vi "Add Headers.vi"(8 "error in (no error)":errorcluster, 10 "headers":cluster{"header":string, "value":string}[](array[cluster]), 11 "HttpHeaders_NET in":refnum<class "HttpHeaders_NET.lvclass">) -> (0 "error out":errorcluster, 3 "HttpHeaders_NET out":refnum<class "HttpHeaders_NET.lvclass">)   [LabVIEW 2018, in "HttpClient_NET.lvlib" / "HttpHeaders_NET.lvclass"]
doc: "<b> </b> <b> </b>\nHttpClient_NET\nJustin Young - Viviota\nCopyright (c) 2021\nLicense: BSD"
uses:
  HttpHeaders_NET.lvclass
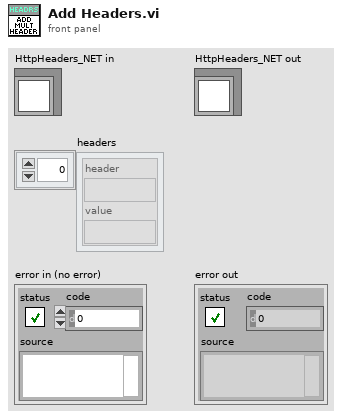
[diagram p1: front panel]
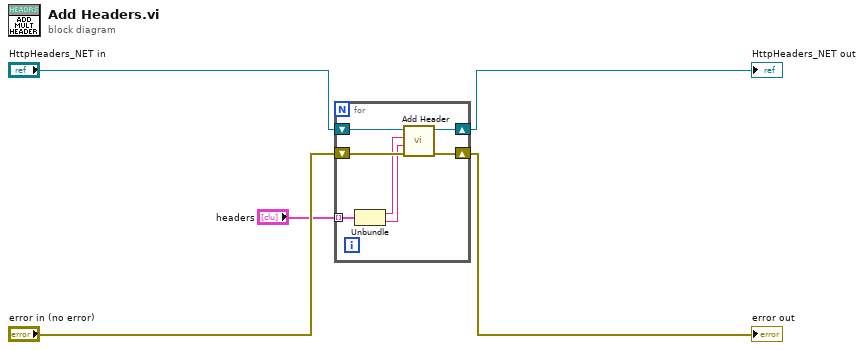
[diagram p0: block diagram]
diagram:
  n1 = for {
    tunnel: "headers" -> [w11] mode=indexing
    shift-right: [w8] -> w4
    shift-left: "HttpHeaders_NET in" -> [w6]
    shift-right: [w7] -> w2
    shift-left: "error in (no error)" -> [w12]
    n2 = Unbundle(w11) -> ("header"=w10:string, "value"=w9:string)
    n3 = call-dynamic "Add Header.vi"("error in (no error)"=w12, "Value"=w9, "Name"=w10, "HTTPHeaders_NET in"=w6) -> ("error out"=w7:errorcluster, "HTTPHeaders_NET out"=w8:refnum<class "HttpHeaders_NET.lvclass">)  [unwired: 6 in]
  }
  "error out" <- w2
  "HttpHeaders_NET out" <- w4
